vi "GetMDPtrQueue.vi"(8 "error in (no error)":errorcluster, 11 "MemoryLength":i32) -> (0 "error out":errorcluster, 2 "Total MDPtrQueue":T1, 3 "MDPtrQueue":T1)   [LabVIEW 2017, in "MDPtr.lvlib" / "MDPtrMgr.lvclass"]
uses:
  MDPtrMgr.lvclass
  MDPtr TypeDef/MDPtr Queue.ctl
  MDPtr TypeDef/MDPtr.ctl
  MDPtr.lvlib
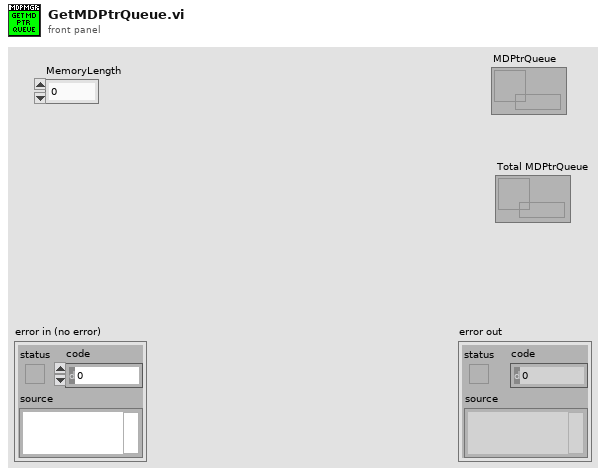
[diagram p1: front panel]
types:
  T1 = typedef "MDPtr.lvlib/MDPtr Queue.ctl" = refnum<queue>
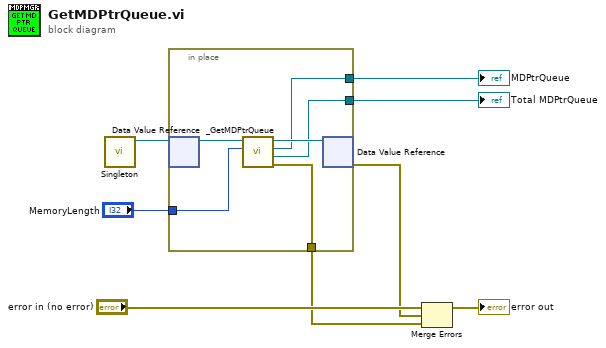
[diagram p0: block diagram]
diagram:
  n1 = call "Singleton.vi"() -> ("MDPtrMgrDVR"=w8:refnum<data-value>)  [unwired: 9 in, 2 out]
  n2 = in-place {
    in-place-border: [w12] -> w4
    in-place-border: "MemoryLength" -> [w11]
    in-place-border: [w10] -> w2
    in-place-border: [w9] -> w1
    n3 = in-place-dvr #1(w8) -> (w14:refnum<class "MDPtrMgr.lvclass">)  [unwired: 1 out]
    n4 = call "_GetMDPtrQueue.vi"("MemoryLength"=w11, "MDPtrMgr in"=w14) -> ("error out"=w12:errorcluster, "Total MDPtrQueue"=w9:T1, "MDPtrQueue"=w10:T1, "MDPtrMgr out"=w13:refnum<class "MDPtrMgr.lvclass">)  [unwired: 6 in]
    n5 = in-place-dvr #1(w13) -> (w5:errorcluster)  [unwired: 1 out]
  }
  "MDPtrQueue" <- w2
  "Total MDPtrQueue" <- w1
  n6 = Merge Errors("error in (no error)", w5, w4) -> (→"error out":errorcluster)
